vi "EscribirVoltaje.vi"(3 "Boolean":bool, 4 "cluster":T1, 5 "data":dbl) -> (0 "Boolean 2":bool, 1 "Cluster":T1, 2 "error out":errorcluster)   [LabVIEW 2017]
uses:
  <vilib>/DAQmx/write.llb/DAQmx Write (Analog DBL 1Chan 1Samp).vi
  <vilib>/DAQmx/miscellaneous.llb/DAQmx Fill In Error Info.vi
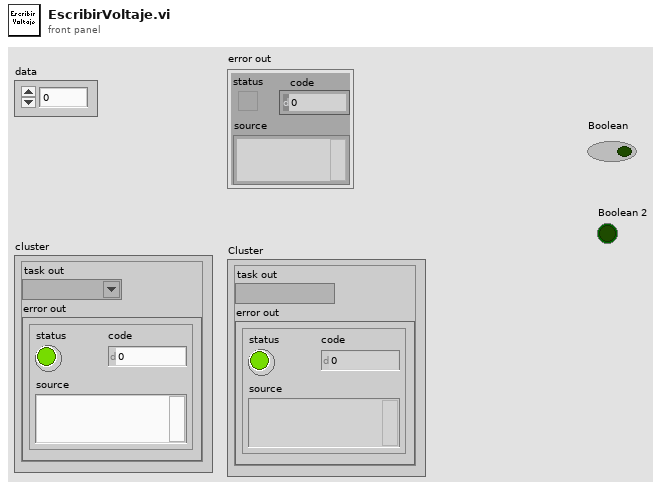
[diagram p1: front panel]
types:
  T1 = cluster{"task out":refnum<k21>, "error out":errorcluster}
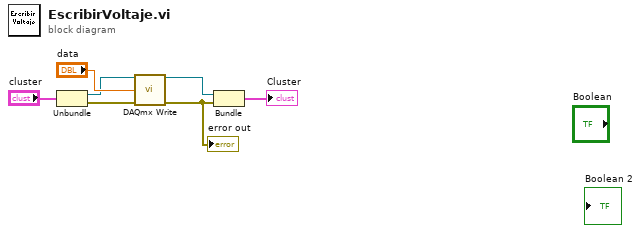
[diagram p0: block diagram]
diagram:
  n1 = Unbundle("cluster") -> ("task out"=w1:refnum<k21>, "error out"=w3:errorcluster)
  n2 = call-poly <vilib>:"DAQmx Write.vi"("task/channels in"=w1, "data"="data", "error in"=w3) -> ("task out"=w4:refnum<k21>, "error out"=w5:errorcluster)  [unwired: 10 in, 1 out]
  "error out" <- w5
  n3 = Bundle("task out"=w4, "error out"=w5) -> (→"Cluster":T1)  [unwired: 1 in]
